vi "automatic_step_address.vi"(7 "transition_queue":refnum<queue>, 8 "error in (no error)":errorcluster, 10 "data":variant, 11 "recipe_data":variant) -> (0 "error out":errorcluster)   [LabVIEW 2015, in "lv-recipe-machine.lvlib" / "example_02.lvlib"]
uses:
  example_02.lvlib
  public/_controls/transition.ctl
  _controls/customer.ctl
  lv-recipe-machine.lvlib
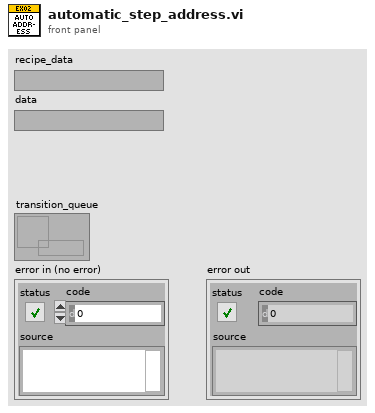
[diagram p1: front panel]
types:
  T1 = typedef "lv-recipe-machine.lvlib/example_02.lvlib/customer.ctl" = cluster{"first_name":string, "last_name":string, "address_1":string, "address_2":string, "city":string, "state":string, "zip_code":string}
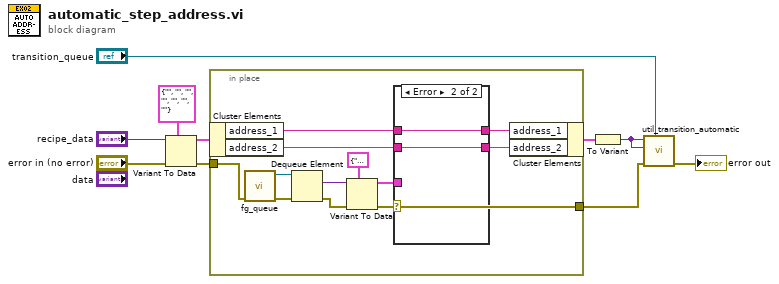
[diagram p0: block diagram]
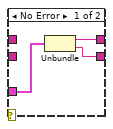
[diagram p2: hidden frame]
diagram:
  n1 = Variant To Data(error in="error in (no error)", type=T1 {"first_name"="", "last_name"="", "address_1"="", "address_2"="", "city"="", "state"="", "zip_code"=""} ("customer"), Variant="recipe_data") -> (data=w5:T1, error out=w2:errorcluster)
  n2 = in-place {
    in-place-border: w2 -> [w20]
    in-place-border: [w17] -> w1
    n3 = in-place-cluster #1(w5) -> ("address_1"=w18:string, "address_2"=w14:string)
    n4 = call "fg_queue.vi"("error in (no error)"=w20) -> ("error out"=w21:errorcluster, "queue out"=w22:refnum<queue>)  [unwired: 9 in]
    n5 = Dequeue Element(queue=w22, error in (no error)=w21) -> (element=w11:variant, error out=w19:errorcluster)  [unwired: 1 in, 2 out]
    n6 = Variant To Data(error in=w19, type=cluster{string, string} {"", ""}, Variant=w11) -> (data=w16:cluster{string, string}, error out=w17:errorcluster)
    n7 = case shown="Error" w17 {
      tunnel: w18 -> [_ w27]
      tunnel: w16 -> [w25 _]
      tunnel: [w24 w27] -> w15
      tunnel: w14 -> [_ w26]
      tunnel: [w23 w26] -> w12
      frame No Error {
        n8 = Unbundle(w25) -> (w24:string, w23:string)
      }
      frame Error {
      }
    }
    n9 = in-place-cluster #1("address_1"=w15, "address_2"=w12) -> (w4:T1)
  }
  n10 = To Variant(anything=w4) -> (Variant=w3:variant)
  n11 = call "util_transition_automatic.vi"("transition_queue"="transition_queue", "error in (no error)"=w1, "data"=w3, "recipe_data"=w3) -> ("error out"=→"error out":errorcluster)  [unwired: 7 in]
